vi "Kaelus SWI Release.vi"(7 "Kaelus SWI":T1, 8 "error in (no error)":errorcluster, 11 "DAQmx Dev Name (SWModule)":string) -> (0 "error out":errorcluster {"code" format="%.0x"})   [LabVIEW 2011]
uses:
  TypeDefs/Kaelus SWI Instrument Info.ctl
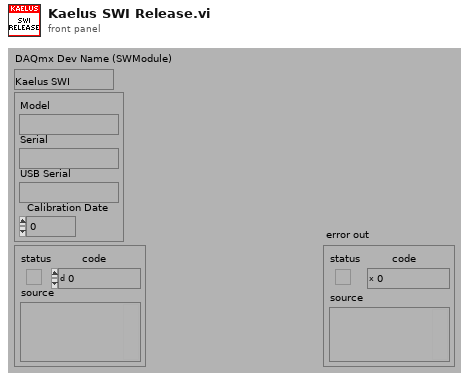
[diagram p1: front panel]
types:
  T1 = typedef "Kaelus SWI Instrument Info.ctl" = cluster{"Model":string, "Serial":string, "USB Serial":string, "Calibration Date":dbl}
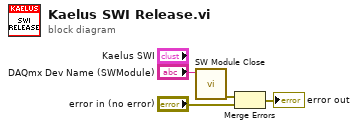
[diagram p0: block diagram]
diagram:
  n1 = call "SW Module Close.vi"("DAQmx Dev Name"="DAQmx Dev Name (SWModule)") -> ("error out"=w3:errorcluster)  [unwired: 6 in]
  n2 = Merge Errors(w3, "error in (no error)") -> (→"error out":errorcluster)
